vi "FormatToObject.vi"(11 "Properties":string[](array[string])) -> (3 "Formatted string":string)   [LabVIEW 2017, in "JsonFormatter.lvlib"]
uses:
  JsonFormatter.lvlib
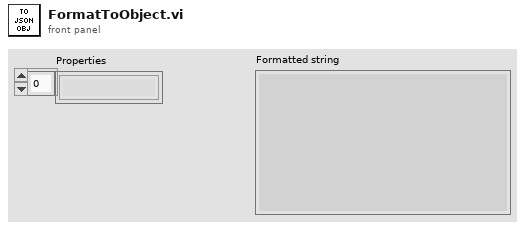
[diagram p1: front panel]
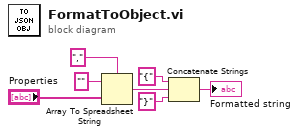
[diagram p0: block diagram]
diagram:
  n1 = Array To Spreadsheet String(delimiter (Tab)=",", array="Properties", 3:"" ("format string")) -> (spreadsheet string=w4:string)
  n2 = Concatenate Strings("{" ("string"), w4, "}" ("string")) -> (→"Formatted string":string)
